vi "optionsMOD.vi"() -> ()   [LabVIEW 2011]
panel:
  in  "Radio Buttons":T1(radio)
  in  "stop":bool
  out "String":string
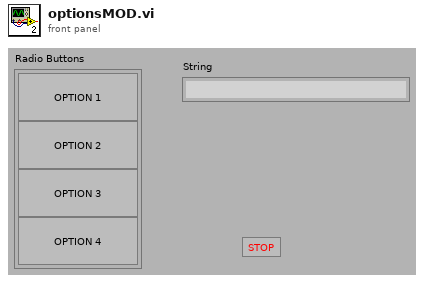
[diagram p1: front panel]
types:
  T1 = enum32{"No Selection", "option 1", "option 2", "option 3", "option 4"}
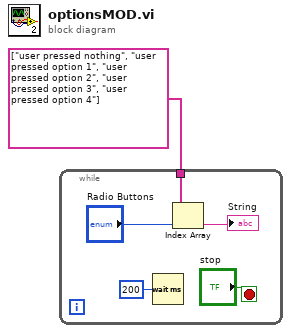
[diagram p0: block diagram]
diagram:
  n1 = while {
    tunnel: string[] ["user pressed nothing", "user pressed option 1", "user pressed option 2", "user pressed option 3", "user pressed option 4"] -> [w3]
    stop <- "stop" stop-if-true
    n2 = Wait (ms)(milliseconds to wait=u32 200) -> ()  [unwired: 1 out]
    n3 = Index Array(array=w3, index="Radio Buttons") -> (element=→"String":string)
  }
